vi "WriteEvtSignalRequest.vi"(8 "error in (no error)":errorcluster, 10 "EvtSignal":dbl[][](array[numeric]), 11 "ModuleID":i32) -> (0 "error out":errorcluster)   [LabVIEW 2014, in "SamplerPlugins.lvlib" / "Simulation.lvclass"]
uses:
  Simulation.lvclass
  SamplerModule/Protected/clEventType.ctl
  <vilib>/Utility/error.llb/Error Cluster From Error Code.vi
  <vilib>/ErrorRing/Error Ring.xnode
  SamplerModule/SamplerModule.lvlib
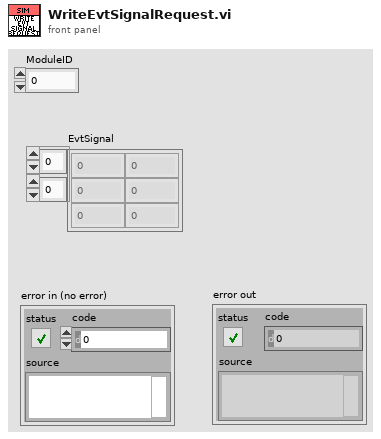
[diagram p1: front panel]
types:
  T1 = typedef "SamplerModule.lvlib/clRequestEvents.ctl" = cluster{"StopRequest":refnum<user-event>, "PathToINI":refnum<user-event>, " LoadPlugin":refnum<user-event>, "ConfigMeasurement":refnum<user-event>, "Read":refnum<user-event>, "GetReading":refnum<user-event>, "InitializeDevice":refnum<user-event>, "ResetRequest":refnum<user-event>, "AbortRequest":refnum<user-event>, "FetchRequest":refnum<user-event>, "InitiateRequest":refnum<user-event>, "ConfigTrigger":refnum<user-event>, "IsOverRange":refnum<user-event>, "ConfigACBandwidth":refnum<user-event>, "ConfigFreqVoltRange":refnum<user-event>, "ConfigMeasCompDest":refnum<user-event>, "FetchMultiPoint":refnum<user-event>, "ReadMultiPoint":refnum<user-event>, "ConfigMultiPoint":refnum<user-event>, "GetMultiPointReading":refnum<user-event>, "InitiateMultiPoint":refnum<user-event>, "ShowPanel":refnum<user-event>, "WriteMultiPointParams":refnum<user-event>, "EvtSignal":refnum<user-event>}
  T2 = typedef "SamplerModule.lvlib/clEventType.ctl" = cluster{"ModuleID":i32, "Data":variant}
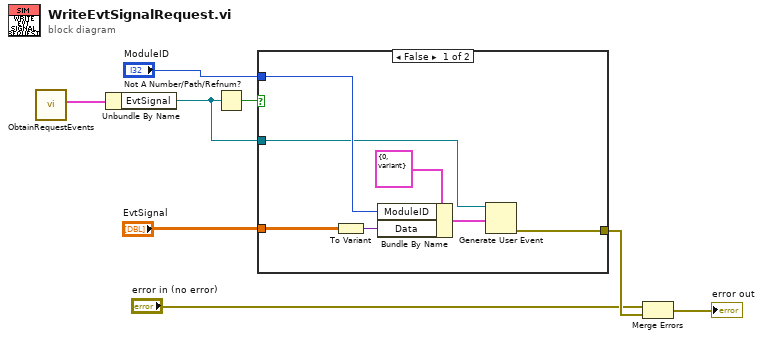
[diagram p0: block diagram]
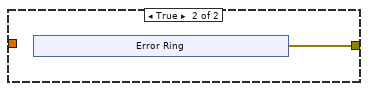
[diagram p2: hidden frame]
diagram:
  n1 = call "ObtainRequestEvents.vi"() -> ("SamplerRequests"=w8:T1)  [unwired: 10 in, 1 out]
  n2 = Unbundle By Name(w8) -> ("EvtSignal"=w6:refnum<user-event>)
  n3 = Not A Number/Path/Refnum?(number/path/refnum=w6) -> (NaN/Path/Refnum?=w7:bool)
  n4 = case shown="False" w7 {
    tunnel: w6 -> [w12 _]
    tunnel: "ModuleID" -> [w14 _]
    tunnel: [w11 w16] -> w3
    tunnel: "EvtSignal" -> [w9 _]
    frame False {
      n5 = To Variant(anything=w9) -> (Variant=w10:variant)
      n6 = Bundle By Name(cluster=T2 {"ModuleID"=0, "Data"=variant} ("clEventType"), "ModuleID"=w14, "Data"=w10) -> (w13:T2)
      n7 = Generate User Event(user event=w12, event data cluster=w13) -> (error out=w11:errorcluster)  [unwired: 2 in, 1 out]
    }
    frame True {
      n8 = xnode "Error Ring"() -> ("error out"=w16:errorcluster)
    }
  }
  n9 = Merge Errors("error in (no error)", w3) -> (→"error out":errorcluster)
